vi "SWEEP 1.vi"(8 "点数":dbl, 9 "终止频率":dbl, 10 "起始频率":dbl, 11 "微波源":refnum<visa-resource-name>="USB0::0x03EB::0xAFFF::341-0A3100002-0514::INSTR" caption="串口选择") -> ()   [LabVIEW 2018]
panel:
  out "连接的字符串":string
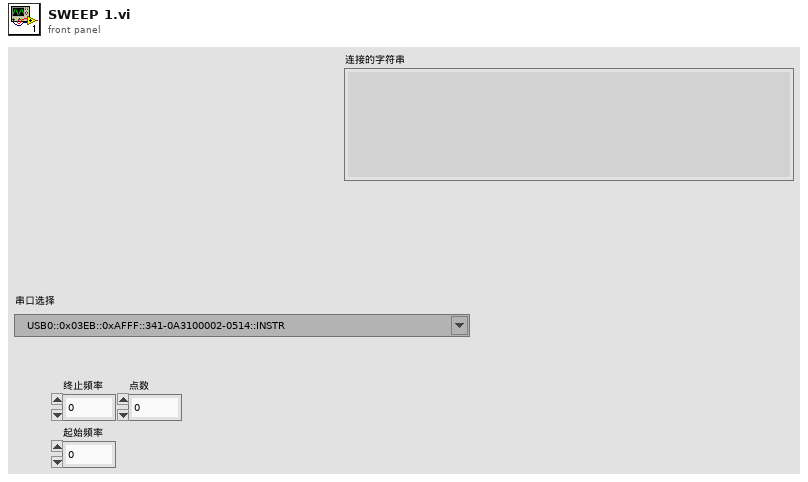
[diagram p1: front panel]
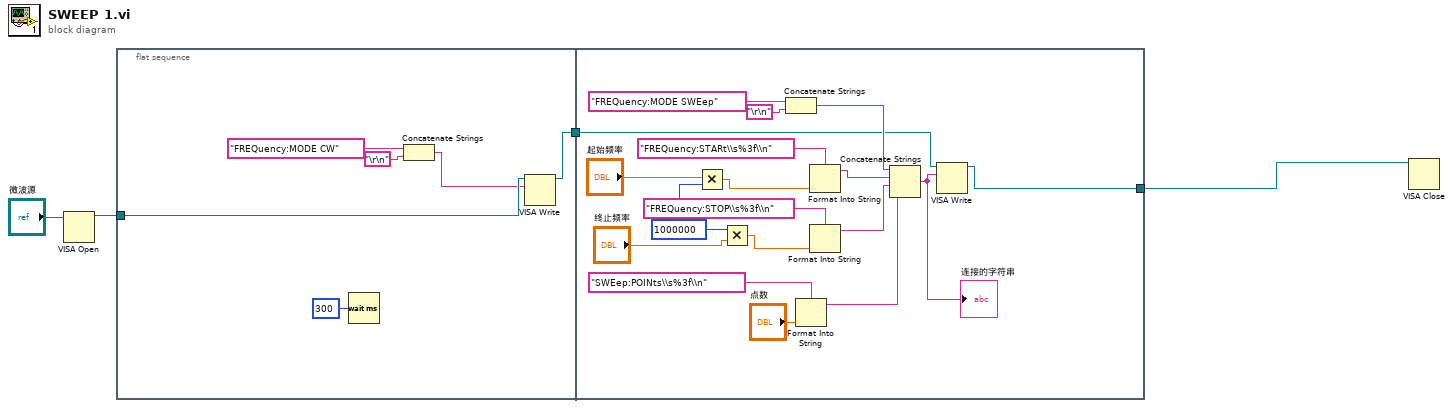
[diagram p0: block diagram]
diagram:
  n1 = VISA Open(VISA resource name="微波源") -> (VISA resource name=w3:refnum<visa-resource-name>)  [unwired: 4 in, 1 out]
  n2 = flat-sequence {
    tunnel: w3 -> [w10]
    tunnel: [w6] -> w1
    tunnel: [w17] -> w2
    tunnel: w1 -> [w18]
    frame #0 {
      n3 = Wait (ms)(milliseconds to wait=u32 300 ("等待时间（毫秒）")) -> ()  [unwired: 1 out]
      n4 = Concatenate Strings("FREQuency:MODE CW" ("格式字符串"), "\r\n") -> (w7:string)
      n5 = VISA Write(VISA resource name=w10, write buffer=w7) -> (VISA resource name out=w6:refnum<visa-resource-name>)  [unwired: 1 in, 2 out]
    }
    frame #1 {
      w13 = 1000000
      n6 = Multiply(x="起始频率", y=w13) -> (x*y=w12:dbl)
      n7 = Multiply(x=w13, y="终止频率") -> (x*y=w15:dbl)
      n8 = Concatenate Strings("FREQuency:MODE SWEep" ("格式字符串"), "\r\n") -> (w23:string)
      n9 = Format Into String(format string="SWEep:POINts\\s%3f\\n" ("格式字符串"), "点数") -> (resulting string=w20:string)  [unwired: 2 in, 1 out]
      n10 = Format Into String(format string="FREQuency:STARt\\s%3f\\n" ("格式字符串"), w12) -> (resulting string=w22:string)  [unwired: 2 in, 1 out]
      n11 = Format Into String(format string="FREQuency:STOP\\s%3f\\n" ("格式字符串"), w15) -> (resulting string=w21:string)  [unwired: 2 in, 1 out]
      n12 = Concatenate Strings(w23, w22, w21, w20) -> (w19:string)
      "连接的字符串" <- w19
      n13 = VISA Write(VISA resource name=w18, write buffer=w19) -> (VISA resource name out=w17:refnum<visa-resource-name>)  [unwired: 1 in, 2 out]
    }
  }
  n14 = VISA Close(VISA resource name=w2) -> ()  [unwired: 1 in, 1 out]
